vi "MultRRTPlan.vi"(10 "IA State":T6={"our_robots"=[], "enemy_robots"=[], "balls"=[], "geometry"={"field_length"=0, "field_width"=0, "goal_width"=0, "goal_depth"=0, "center_circle_radius"=0, "defense_width"=0, "defense_depth"=0, "free_kick_from_defense_dist"=0, "penalty_spot_from_field_line_dist"=0, "penalty_line_from_spot_dist"=0, "half_moon_depth"=0, "half_moon_width"=0}, "IA Judge"={"stage"="", "command"="", "our_goalie_id"=0.0, "enemy_goalie_id"=0.0, "command enum"=enum."Halt", "Time"=enum."Azul"}, "Received Timestamp"=timestamp(0 s since 1904-01-01), "Events"={"Touch"=FALSE, "Ball out"=FALSE, "id touch"=0.0, "Ball out of \nVision"=FALSE, "Ball inside \nGoalie area"=FALSE, "Robot not responding"=FALSE, "Robots responding status"=[1.0, 1.0, 1.0, 1.0, 1.0, 1.0], "Enemy Ball \nPossession"=FALSE, "Pass State"=FALSE, "id end of pass"=0.0, "Kick"=FALSE, "Id ini Possession"=0.0, "Ball Possesion"=FALSE, "Id Possesion"=0.0}}, 11 "Robot":T1={"id"=0, "function"=enum."Attacker", "x"=0.0, "y"=0.0, "orientation"=0.0, "v_tangent"=0.0, "v_normal"=0.0, "v_ang"=0.0, "kick_x"=0.0, "kick_z"=0.0, "dribble"=FALSE, "Timestamp"=timestamp(0 s since 1904-01-01), "estimatives"={"est_v_tangent"=0.0, "est_v_normal"=0.0, "est_vx"=0.0, "est_vy"=0.0, "Pos Robot Est"=[]}, "dest_x_kick"=0.0, "dest_y_kick"=0.0, "Gap Coord"=[], "States"=enum."GoToTangent", "Path "=[], "Path  Smooth"=[], "Dest"=[]}) -> (2 "Robot Out":T1={"id"=0, "function"=enum."Attacker", "x"=0.0, "y"=0.0, "orientation"=0.0, "v_tangent"=0.0, "v_normal"=0.0, "v_ang"=0.0, "kick_x"=0.0, "kick_z"=0.0, "dribble"=FALSE, "Timestamp"=timestamp(0 s since 1904-01-01), "estimatives"={"est_v_tangent"=0.0, "est_v_normal"=0.0, "est_vx"=0.0, "est_vy"=0.0, "Pos Robot Est"=[]}, "dest_x_kick"=0.0, "dest_y_kick"=0.0, "Gap Coord"=[], "States"=enum."GoToTangent", "Path "=[], "Path  Smooth"=[], "Dest"=[]})   [LabVIEW 2017]
uses:
  Core/AI Robot.ctl
  Intel/Functions Enum.ctl
  Intel/AttackerStates.ctl
  PathDests.ctl
  PathDest.ctl
  Core/AI Input.ctl
  Core/AI Ball.ctl
  Core/Field Size.ctl
  Core/AI Judge.ctl
  Intel/Command Enum.ctl
  Util/Events/Events.ctl
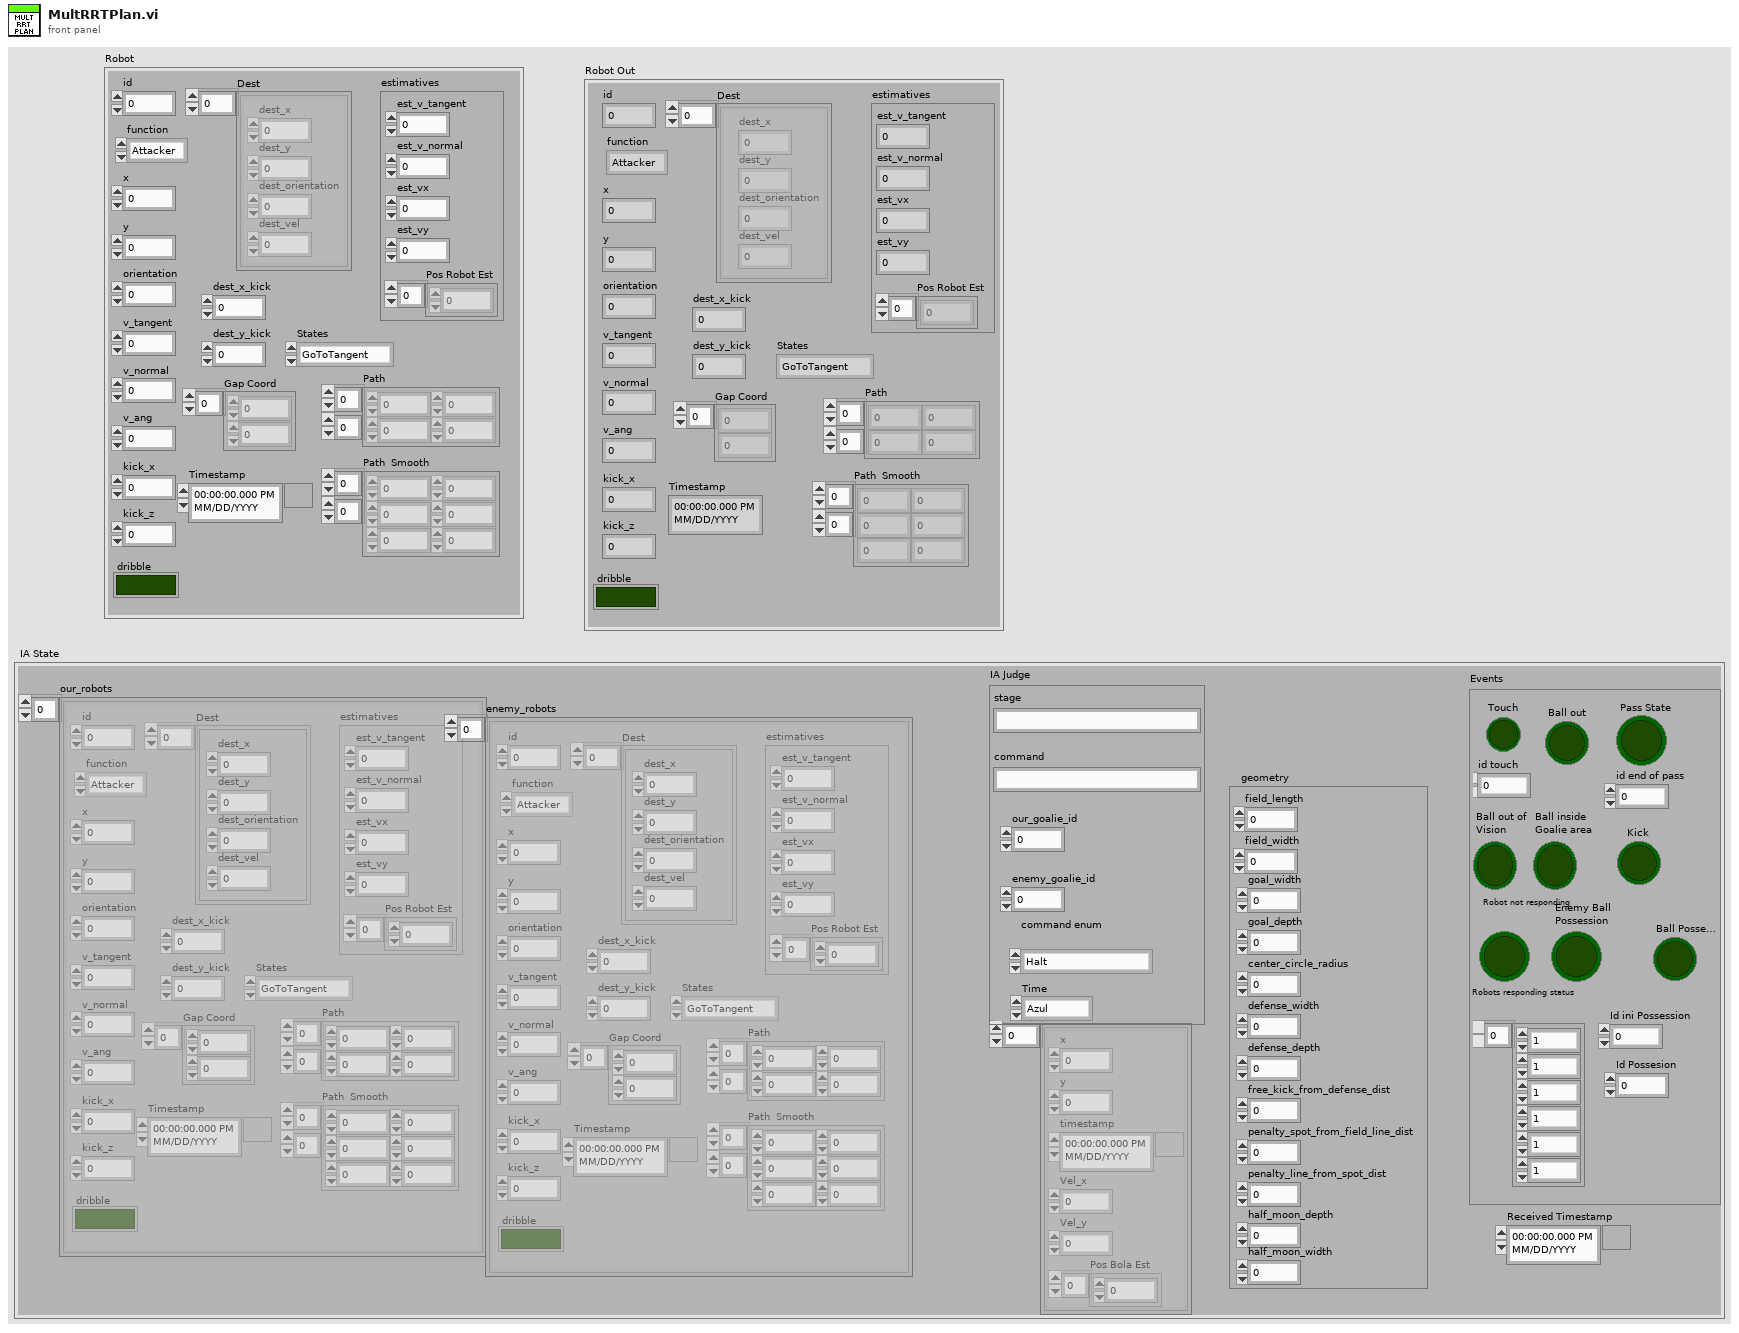
[diagram p1: front panel]
types:
  T1 = typedef "AI Robot.ctl" = cluster{"id":u32, "function":T2, "x":dbl, "y":dbl, "orientation":dbl, "v_tangent":dbl, "v_normal":dbl, "v_ang":dbl, "kick_x":dbl, "kick_z":dbl, "dribble":bool, "Timestamp":timestamp, "estimatives":cluster{"est_v_tangent":dbl, "est_v_normal":dbl, "est_vx":dbl, "est_vy":dbl, "Pos Robot Est":dbl[]}, "dest_x_kick":dbl, "dest_y_kick":dbl, "Gap Coord":dbl[], "States":T3, "Path ":dbl[][], "Path  Smooth":dbl[][], "Dest":T4}
  T2 = typedef "Functions Enum.ctl" = enum16{"Attacker", "Goalie", "Defender", "Striker", "Goto 0", "Dummy", "Kicker", "ZigZag"}
  T3 = typedef "AttackerStates.ctl" = enum16{"Pass", "GoToTangent", "BallGetting", "GoToKick", ""}
  T4 = typedef "PathDests.ctl" = T5[]
  T5 = typedef "PathDest.ctl" = cluster{"dest_x":dbl, "dest_y":dbl, "dest_orientation":dbl, "dest_vel":dbl}
  T6 = typedef "AI Input.ctl" = cluster{"our_robots":T1[], "enemy_robots":T1[], "balls":T7[], "geometry":T8, "IA Judge":T9, "Received Timestamp":timestamp, "Events":T11}
  T7 = typedef "AI Ball.ctl" = cluster{"x":dbl, "y":dbl, "timestamp":timestamp, "Vel_x":dbl, "Vel_y":dbl, "Pos Bola Est":dbl[]}
  T8 = typedef "Field Size.ctl" = cluster{"field_length":u32, "field_width":u32, "goal_width":u32, "goal_depth":u32, "center_circle_radius":u32, "defense_width":u32, "defense_depth":u32, "free_kick_from_defense_dist":u32, "penalty_spot_from_field_line_dist":u32, "penalty_line_from_spot_dist":u32, "half_moon_depth":u32, "half_moon_width":u32}
  T9 = typedef "AI Judge.ctl" = cluster{"stage":string, "command":string, "our_goalie_id":dbl, "enemy_goalie_id":dbl, "command enum":T10, "Time":enum16{"Azul", "Amarelo"}}
  T10 = typedef "Command Enum.ctl" = enum16{"Halt", "Stop", "Force Start", "PKA Normal Start", "Prepare Kickoff Ally", "PKE Normal Start", "Prepare Kickoff Enemy", "Prepare Penalty Ally", "PPA Normal Start", "Prepare Penalty Enemy", "PPE Normal Start", "Direct Free Enemy", "Direct Free Ally", "Indirect Free Enemy", "Indirect Free Ally", "Timeout Enemy", "Timeout Ally", "Goal Enemy", "Goal Ally", "Ball Placement Enemy", "Ball Placement Ally", "Normal Half Time", "Extra Time Break", "Extra Half Time", "None", "Post Game"}
  T11 = typedef "Events.ctl" = cluster{"Touch":bool, "Ball out":bool, "id touch":dbl, "Ball out of \nVision":bool, "Ball inside \nGoalie area":bool, "Robot not responding":bool, "Robots responding status":dbl[], "Enemy Ball \nPossession":bool, "Pass State":bool, "id end of pass":dbl, "Kick":bool, "Id ini Possession":dbl, "Ball Possesion":bool, "Id Possesion":dbl}
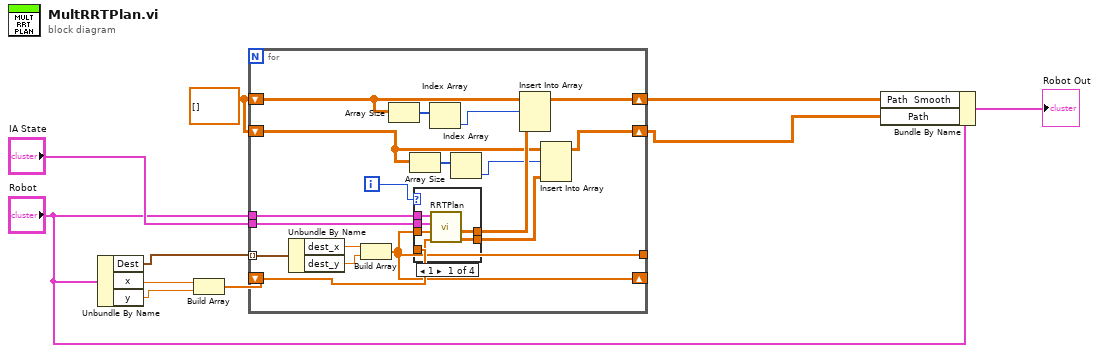
[diagram p0: block diagram]
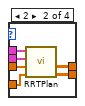
[diagram p2: hidden frame]
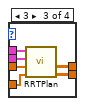
[diagram p3: hidden frame]
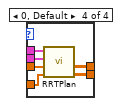
[diagram p4: hidden frame]
diagram:
  w5 = dbl[][] [] ("Path")
  n1 = Unbundle By Name("Robot") -> ("Dest"=w3:T4, "x"=w10:dbl, "y"=w9:dbl)
  n2 = Build Array(w10, w9) -> (w6:dbl[])
  n3 = for {
    tunnel: "Robot" -> [w27]
    tunnel: "IA State" -> [w28]
    shift-right: [w21] -> w1
    shift-left: w5 -> [w20]
    tunnel: w3 -> [w26] mode=indexing
    shift-right: [w17] -> _
    shift-left: w6 -> [w23]
    tunnel: [w17] -> _
    shift-right: [w13] -> w2
    shift-left: w5 -> [w14]
    i -> [w11]
    n4 = Unbundle By Name(w26) -> ("dest_x"=w25:dbl, "dest_y"=w24:dbl)
    n5 = Build Array(w25, w24) -> (w17:dbl[])
    n6 = Array Size(array=w20) -> (size(s)=w19:i32[])
    n7 = Array Size(array=w14) -> (size(s)=w15:i32[])
    n8 = case shown="1" w11 {
      tunnel: w28 -> [w34 w40 w46 w52]
      tunnel: w27 -> [w33 w39 w45 w51]
      tunnel: w23 -> [w32 w38 w44 w50]
      tunnel: [w31 w37 w43 w49] -> w22
      tunnel: w17 -> [w30 w36 w42 w48]
      tunnel: [w29 w35 w41 w47] -> w12
      frame 1 {
        n9 = call "RRTPlan.vi"("Initial Pos x,y"=w32, "Dest x,y"=w30, "IA State"=w34, "Robot"=w33) -> ("Path"=w29:dbl[][], "Smooth Path"=w31:dbl[][])  [unwired: 6 in]
      }
      frame 2 {
        n10 = call "RRTPlan.vi"("Initial Pos x,y"=w38, "Dest x,y"=w36, "IA State"=w40, "Robot"=w39) -> ("Path"=w35:dbl[][], "Smooth Path"=w37:dbl[][])  [unwired: 6 in]
      }
      frame 3 {
        n11 = call "RRTPlan.vi"("Initial Pos x,y"=w44, "Dest x,y"=w42, "IA State"=w46, "Robot"=w45) -> ("Path"=w41:dbl[][], "Smooth Path"=w43:dbl[][])  [unwired: 6 in]
      }
      frame 0, Default {
        n12 = call "RRTPlan.vi"("Initial Pos x,y"=w50, "Dest x,y"=w48, "IA State"=w52, "Robot"=w51) -> ("Path"=w47:dbl[][], "Smooth Path"=w49:dbl[][])  [unwired: 6 in]
      }
    }
    n13 = Index Array(array=w19) -> (element=w18:i32)  [unwired: 1 in]
    n14 = Index Array(array=w15) -> (element=w16:i32)  [unwired: 1 in]
    n15 = Insert Into Array(array=w20, index (row)=w18, new element=w22) -> (w21:dbl[][])  [unwired: 1 in]
    n16 = Insert Into Array(array=w14, index (row)=w16, new element=w12) -> (w13:dbl[][])  [unwired: 1 in]
  }
  n17 = Bundle By Name(cluster="Robot", "Path  Smooth"=w1, "Path"=w2) -> (→"Robot Out":T1)
